vi "write_attributes.vi"(8 "error in (no error)":errorcluster, 10 "attributes":T1, 11 "Ridge in":refnum<class "Ridge.lvclass">) -> (0 "error out":errorcluster, 3 "Ridge out":refnum<class "Ridge.lvclass">)   [LabVIEW 2020, in "Ridge.lvclass"]
uses:
  Ridge.lvclass
  Controls/ridge_attributes.ctl
  Ridge.lvclass/Ridge.ctl
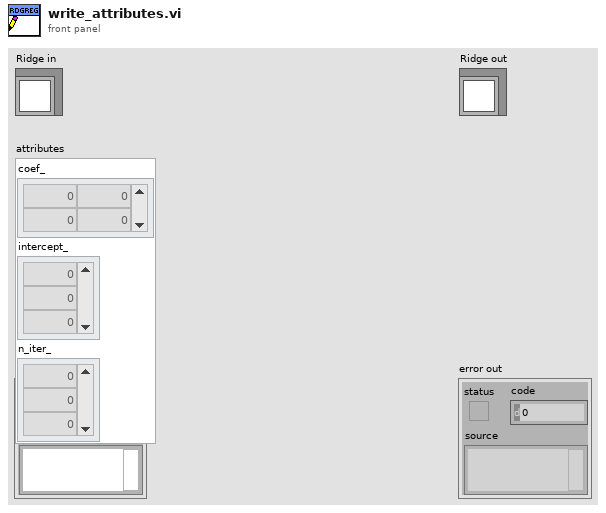
[diagram p1: front panel]
types:
  T1 = typedef "ridge_attributes.ctl" = cluster{"coef_":dbl[][], "intercept_":dbl[], "n_iter_":dbl[]}
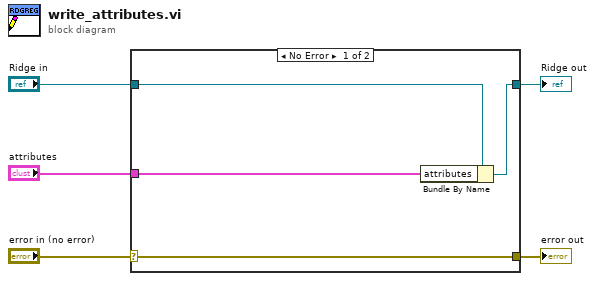
[diagram p0: block diagram]
diagram:
  n1 = case shown="No Error" "error in (no error)" {
    selector: "error in (no error)" -> [w9 w10]
    tunnel: [w9 w10] -> w4
    tunnel: [w7 w11] -> w2
    tunnel: "Ridge in" -> [w8 w11]
    tunnel: "attributes" -> [w6 _]
    frame No Error {
      n2 = Bundle By Name(cluster=w8, "attributes"=w6) -> (w7:refnum<class "Ridge.lvclass">)
    }
    frame Error {
    }
  }
  "error out" <- w4
  "Ridge out" <- w2
